vi "Sql query generator.vi"(7 "Modo":T1, 8 "error in":errorcluster, 10 "Variant":variant) -> (0 "error out":errorcluster, 3 "Query":string)   [LabVIEW 2020]
uses:
  Controles/Sql.ctl
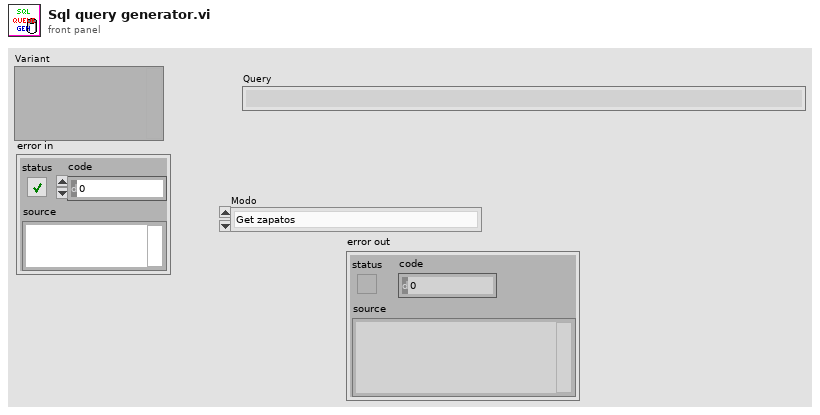
[diagram p1: front panel]
types:
  T1 = typedef "Sql.ctl" = enum16{"Get zapatos", "Insrt Zapatos", "Insrt Elementos", "Borrar Elementos"}
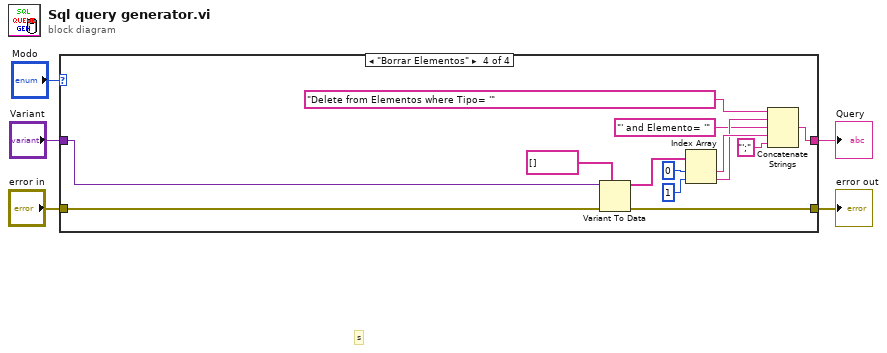
[diagram p0: block diagram]
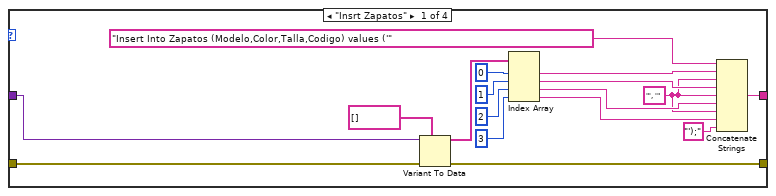
[diagram p2: hidden frame]
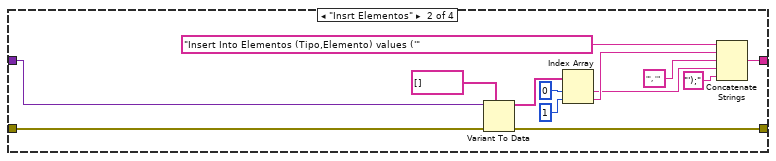
[diagram p3: hidden frame]
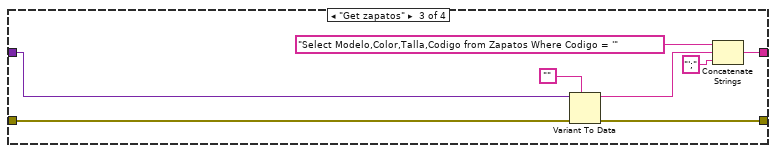
[diagram p4: hidden frame]
diagram:
  # "s"
  n1 = case shown="\"Borrar Elementos\"" "Modo" {
    tunnel: "Variant" -> [w8 w35 w37 w47]
    tunnel: "error in" -> [w19 w34 w43 w46]
    tunnel: [w13 w28 w41 w44] -> w1
    tunnel: [w7 w27 w38 w45] -> w2
    frame "Insrt Zapatos" {
      w16 = "', '" ("string")
      n2 = Variant To Data(error in=w19, type=string[] [], Variant=w8) -> (data=w6:string[], error out=w7:errorcluster)
      n3 = Index Array(array=w6, index #1=0 ("index (row)"), index #2=1 ("disabled index (col)"), index #3=2 ("disabled index (col)"), index #4=3 ("disabled index (col)")) -> (element #1=w21:string, element #2=w20:string, element #3=w17:string, element #4=w15:string)
      n4 = Concatenate Strings("Insert Into Zapatos (Modelo,Color,Talla,Codigo) values ('", w21, w16, w20, w16, w17, w16, w15, "');" ("string")) -> (w13:string)
    }
    frame "Insrt Elementos" {
      n5 = Variant To Data(error in=w34, type=string[] [], Variant=w35) -> (data=w23:string[], error out=w27:errorcluster)
      n6 = Index Array(array=w23, index #1=0 ("index (row)"), index #2=1 ("disabled index (col)")) -> (element #1=w24:string, element #2=w25:string)
      n7 = Concatenate Strings("Insert Into Elementos (Tipo,Elemento) values ('", w25, "', '" ("string"), w24, "');" ("string")) -> (w28:string)
    }
    frame "Get zapatos" {
      n8 = Variant To Data(error in=w43, type="", Variant=w37) -> (data=w36:string, error out=w38:errorcluster)
      n9 = Concatenate Strings("Select Modelo,Color,Talla,Codigo from Zapatos Where Codigo = '", w36, "';" ("string")) -> (w41:string)
    }
    frame "Borrar Elementos" {
      n10 = Variant To Data(error in=w46, type=string[] [], Variant=w47) -> (data=w56:string[], error out=w45:errorcluster)
      n11 = Index Array(array=w56, index #1=0 ("index (row)"), index #2=1 ("disabled index (col)")) -> (element #1=w55:string, element #2=w54:string)
      n12 = Concatenate Strings("Delete from Elementos where Tipo= '", w54, "' and Elemento= '" ("string"), w55, "';" ("string")) -> (w44:string)
    }
  }
  "error out" <- w2
  "Query" <- w1
